vi "__SG_83630L.vi"(0 "PW(dBm)":string="-5", 1 "frq(GHz)":string="12", 2 "GPIB":string="19") -> ()   [LabVIEW 2017]
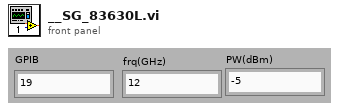
[diagram p1: front panel]
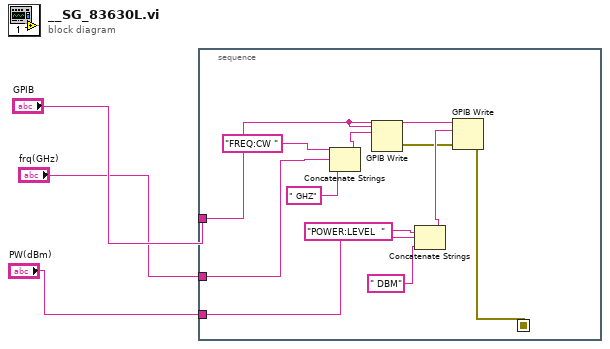
[diagram p0: block diagram]
diagram:
  n1 = stacked-sequence {
    seq-local: [w10] -> [_]
    tunnel: "GPIB" -> [w9]
    tunnel: "frq(GHz)" -> [w8]
    tunnel: "PW(dBm)" -> [w5]
    frame #0 {
      n2 = Concatenate Strings("FREQ:CW ", w8, " GHZ") -> (w13:string)
      n3 = GPIB Write(0:w9, 1:w13) -> (6:w11:errorcluster)  [unwired: 3 in, 1 out]
      n4 = Concatenate Strings("POWER:LEVEL  ", w5, " DBM") -> (w12:string)
      n5 = GPIB Write(0:w9, 1:w12, 3:w11) -> (6:w10:errorcluster)  [unwired: 2 in, 1 out]
    }
  }
